vi "Revision Query Core.vi"(8 "error in (no error)":errorcluster, 11 "IVI_DMM in":refnum<class "IVI_DMM.lvclass">) -> (0 "error out":errorcluster, 1 "Firmware Revision":string, 2 "Driver Revision":string, 3 "IVI_DMM out":refnum<class "IVI_DMM.lvclass">)   [LabVIEW 2015, in "IVI_DMM.lvlib" / "IVI_DMM.lvclass"]
uses:
  IVI_DMM.lvclass
  IVI_DMM.lvclass/IVI_DMM.ctl
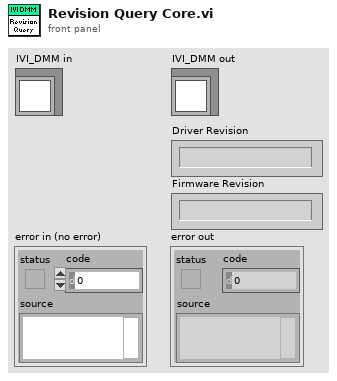
[diagram p1: front panel]
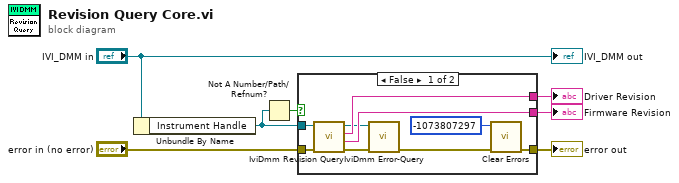
[diagram p0: block diagram]
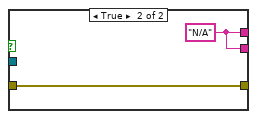
[diagram p2: hidden frame]
diagram:
  n1 = Unbundle By Name("IVI_DMM in") -> ("Instrument Handle"=w2:refnum<k15>)
  n2 = Not A Number/Path/Refnum?(number/path/refnum=w2) -> (NaN/Path/Refnum?=w1:bool)
  n3 = case shown="False" w1 {
    tunnel: "error in (no error)" -> [w16 w18]
    tunnel: [w15 w17] -> w5
    tunnel: [w14 w17] -> w4
    tunnel: [w10 w18] -> w3
    tunnel: w2 -> [w8 _]
    frame False {
      n4 = call <vilib>:"IviDmm Revision Query.vi"("error in (no error)"=w16, "instrument handle"=w8) -> ("error out"=w12:errorcluster, "firmware revision"=w14:string, "instrument driver revision"=w15:string, "instrument handle out"=w13:refnum<k15>)  [unwired: 6 in]
      n5 = call <vilib>:"IviDmm Error-Query.vi"("error in (no error)"=w12, "instrument handle"=w13) -> ("error out"=w11:errorcluster)  [unwired: 6 in, 3 out]
      n6 = call <vilib>:"Clear Errors.vi"("error in (no error)"=w11, "specific error code to clear (0: all)"=-1073807297) -> ("error out"=w10:errorcluster)  [unwired: 4 in, 1 out]
    }
    frame True {
      w17 = "N/A" ("instrument driver revision")
    }
  }
  "error out" <- w3
  "Driver Revision" <- w5
  "Firmware Revision" <- w4
  "IVI_DMM out" <- "IVI_DMM in"
